vi "F Dwf Digital Out Divider Info.vi"(7 "vMax":u32, 8 "error in (no error)":errorcluster, 9 "vMin":u32, 10 "idxChannel":i32, 11 "hdwf":i32) -> (0 "error out":errorcluster, 1 "vMin out":u32, 3 "function return":i32, 5 "vMax out":u32)   [LabVIEW 2024, in "Olasdwf.lvlib"]
doc: "DWFAPI int FDwfDigitalOutDividerInfo(HDWF hdwf, int idxChannel, unsigned int *vMin, unsigned int *vMax);"
uses:
  Olasdwf.lvlib
  Windows/System32/dwf.dll
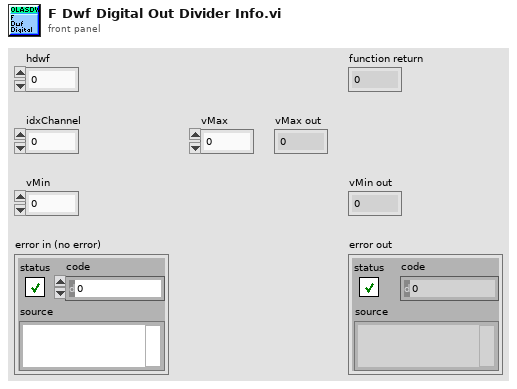
[diagram p1: front panel]
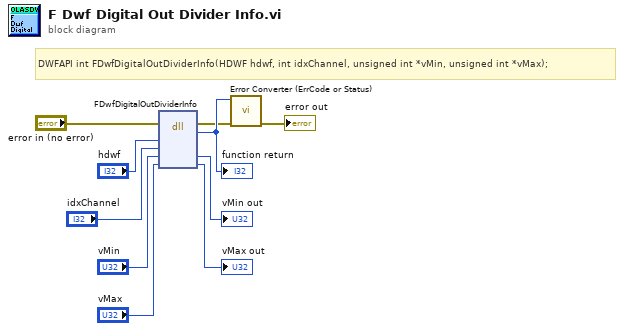
[diagram p0: block diagram]
diagram:
  # "DWFAPI int FDwfDigitalOutDividerInfo(HDWF hdwf, int idxChannel, unsigned int *vMin, unsigned int *vMax);"
  n1 = dll-call lib="/Windows/System32/dwf.*" fn="FDwfDigitalOutDividerInfo"(error in="error in (no error)", "hdwf"="hdwf", "idxChannel"="idxChannel", "vMin"="vMin", "vMax"="vMax") -> (error out=w2:errorcluster, w10:i32, "vMin"=→"vMin out":u32, "vMax"=→"vMax out":u32)  [unwired: 4 in, 1 out]
  "function return" <- w10
  n2 = call "Error Converter (ErrCode or Status).vi"("error in (no error)"=w2, "error code"=w10) -> ("error out"=→"error out":errorcluster)  [unwired: 9 in]
